vi "Trigger Manager Subpanel gRPC Connect Event.vi"(8 "error in (no error)":errorcluster, 11 "CIF_Manager_UI in":refnum<class "CIF_Manager_UI.lvclass">) -> (0 "error out":errorcluster)   [LabVIEW 2021, in "CIF_Manager_UI.lvclass"]
uses:
  CIF_Manager_UI.lvclass
  C:/Program Files/National Instruments/LabVIEW 2021/vi.lib/CIF Foundation/CIF Core/CIFUI/CIF_UI.lvclass
  <vilib>/CIF Foundation/CIF Core/CIFUI/Typedef/New Connection Event Data.ctl
  <vilib>/gRPC/LabVIEW gRPC Library/Shared/grpcId.ctl
  <vilib>/CIF Foundation/CIF Core/CIFUI/CIF_UI.lvclass/CIF_UI.ctl
  <vilib>/CIF Foundation/CIF Core/CIFUI/Accessors/Read Subpanel Events.vi
  <vilib>/CIF Foundation/CIF Core/CIFUI/Accessors/Read Manager gRPC ID.vi
  <vilib>/CIF Foundation/CIF Core/CIFUI/Accessors/Read IP Address.vi
  <vilib>/CIF Foundation/CIF Core/CIFUI/Accessors/Read Connected.vi
  <vilib>/gRPC/LabVIEW gRPC Library/grpc-lvsupport-release.lvlib
  <vilib>/CIF Foundation/CIF Core/CIFUI/CIF_UI.lvclass
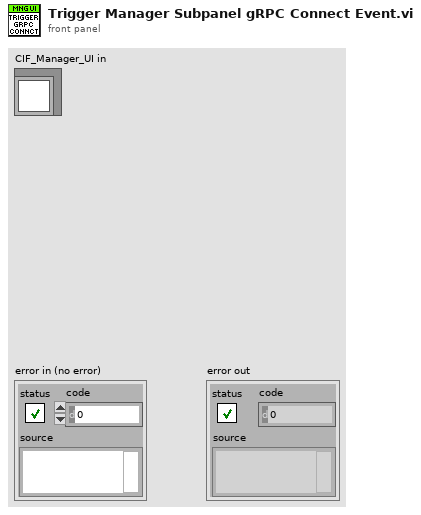
[diagram p1: front panel]
types:
  T1 = typedef "CIF_UI.lvclass/New Connection Event Data.ctl" = cluster{"Manager gRPC ID":T2, "IP Address":string, "Connected":bool}
  T2 = typedef "grpc-lvsupport-release.lvlib/grpcId.ctl" = u64
  T3 = typedef "CIF_UI.lvclass/SubPanel Events.ctl" = cluster{"Clear Local Error":refnum<user-event>, "Shutdown":refnum<user-event>, "gRPC Connection":refnum<user-event>, "Plugin Connection":refnum<user-event>}
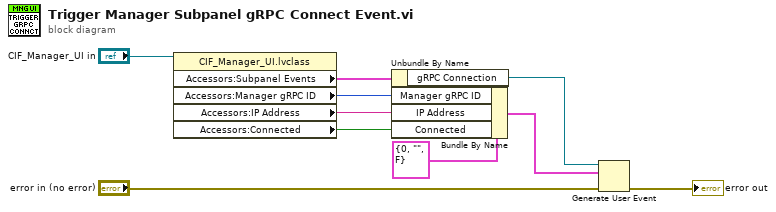
[diagram p0: block diagram]
diagram:
  n1 = property class="CIF_Manager_UI.lvclass"(reference="CIF_Manager_UI in") -> ("Accessors:Subpanel Events"=w8:T3, "Accessors:Manager gRPC ID"=w4:T2, "Accessors:IP Address"=w2:string, "Accessors:Connected"=w1:bool)  [unwired: 1 in, 2 out]
  n2 = Unbundle By Name(w8) -> ("gRPC Connection"=w7:refnum<user-event>)
  n3 = Bundle By Name(cluster=T1 {"Manager gRPC ID"=0, "IP Address"="", "Connected"=FALSE} ("gRPC Connection Data"), "Manager gRPC ID"=w4, "IP Address"=w2, "Connected"=w1) -> (w3:T1)
  n4 = Generate User Event(user event=w7, event data cluster=w3, error in="error in (no error)") -> (error out=→"error out":errorcluster)  [unwired: 1 in, 1 out]
